vi "Event Handle Loop_Mouse Down.vi"(8 "error in (no error)":errorcluster, 10 "Coords":T1, 11 "QMenu Class in":refnum<class "QMenu Class.lvclass">) -> (0 "error out":errorcluster, 3 "QMenu Class out":refnum<class "QMenu Class.lvclass">)   [LabVIEW 2020, in "QTab.lvlib" / "QMenu Class.lvclass"]
uses:
  QMenu Class.lvclass
  <vilib>/Utility/miscctls.llb/LVPoint32TypeDef.ctl
  QMenu Class.lvclass/QMenu Class.ctl
  Read Total Button Count.vi
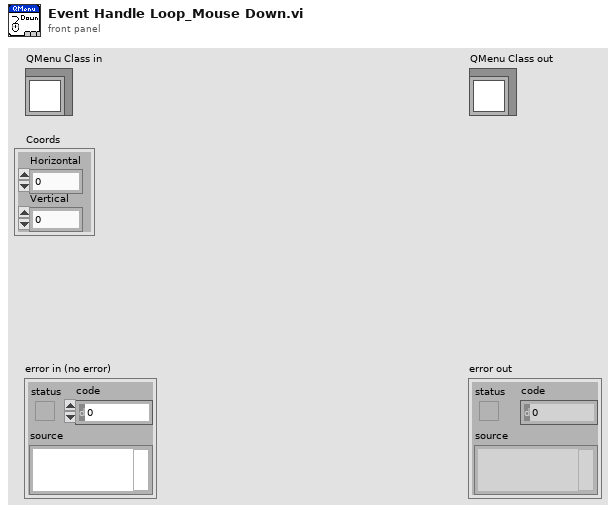
[diagram p1: front panel]
types:
  T1 = typedef "LVPoint32TypeDef.ctl" = cluster{"Horizontal":i32, "Vertical":i32}
  T2 = typedef "QTab.lvlib/QMenu Class.lvclass/Button Attribute.ctl" = cluster{"Label":string, "Button Text":string, "Closable":bool, "Draggable":bool}
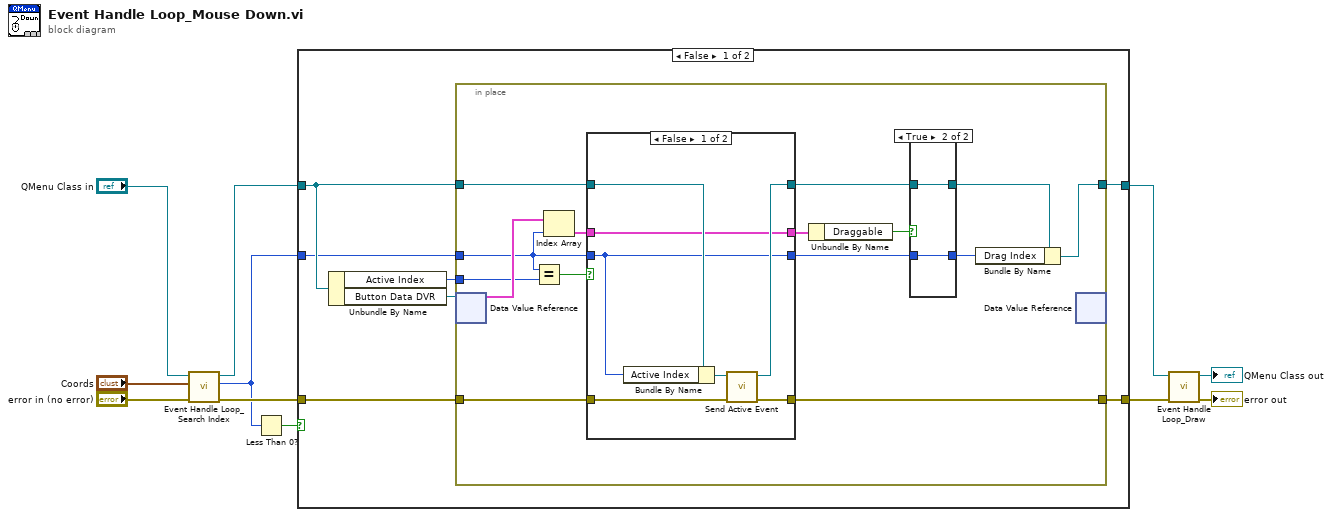
[diagram p0: block diagram]
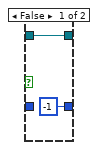
[diagram p2: hidden frame]
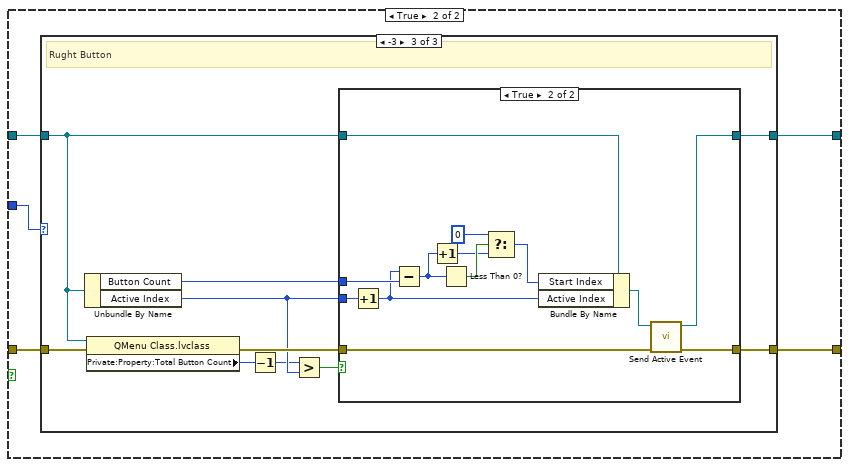
[diagram p4: hidden frame]
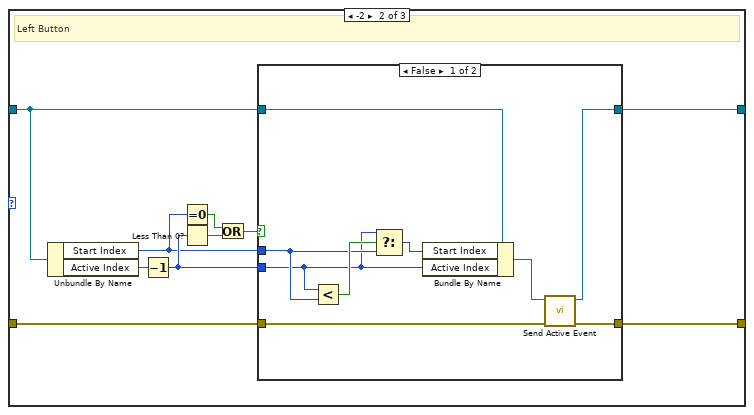
[diagram p6: hidden frame]
diagram:
  n1 = call "Event Handle Loop_Search Index.vi"("error in (no error)"="error in (no error)", "Coords"="Coords", "QMenu Class in"="QMenu Class in") -> ("error out"=w11:errorcluster, "Index"=w9:i32, "QMenu Class out"=w2:refnum<class "QMenu Class.lvclass">)  [unwired: 6 in]
  n2 = Less Than 0?(x=w9) -> (x < 0?=w3:bool)
  n3 = case shown="False" w3 {
    tunnel: w2 -> [w17 w51]
    tunnel: w9 -> [w13 w52]
    tunnel: [w14 w49] -> w1
    tunnel: w11 -> [w18 w53]
    tunnel: [w16 w50] -> w6
    frame False {
      n4 = Unbundle By Name(w17) -> ("Active Index"=w12:i32, "Button Data DVR"=w15:refnum<data-value>)
      n5 = in-place {
        in-place-border: w13 -> [w25]
        in-place-border: w18 -> [w33]
        in-place-border: w17 -> [w31]
        in-place-border: [w22] -> w16
        in-place-border: [w19] -> w14
        in-place-border: w12 -> [w24]
        n6 = in-place-dvr #1(w15) -> (w30:T2[])  [unwired: 1 out]
        n7 = Equal?(x=w25, y=w24) -> (x = y?=w32:bool)
        n8 = Index Array(array=w30, index=w25) -> (element=w29:T2)
        n9 = case shown="False" w32 {
          tunnel: w33 -> [w43 w48]
          tunnel: w31 -> [w44 w47]
          tunnel: [w40 w47] -> w26
          tunnel: [w41 w48] -> w22
          tunnel: w29 -> [w39 w46]
          tunnel: [w39 w46] -> w28
          tunnel: w25 -> [w38 w45]
          tunnel: [w38 w45] -> w23
          frame False {
            n10 = Bundle By Name(cluster=w44, "Active Index"=w38) -> (w42:refnum<class "QMenu Class.lvclass">)
            n11 = call "Send Active Event.vi"("error in (no error)"=w43, "QMenu Class in"=w42) -> ("error out"=w41:errorcluster, "QMenu Class out"=w40:refnum<class "QMenu Class.lvclass">)  [unwired: 8 in]
          }
          frame True {
          }
        }
        n12 = Unbundle By Name(w28) -> ("Draggable"=w27:bool)
        n13 = case shown="True" w27 {
          tunnel: w26 -> [w35 w36]
          tunnel: [w35 w36] -> w21
          tunnel: w23 -> [_ w37]
          tunnel: [-1 ("Index") w37] -> w20
          frame False {
          }
          frame True {
          }
        }
        n14 = Bundle By Name(cluster=w21, "Drag Index"=w20) -> (w19:refnum<class "QMenu Class.lvclass">)
        n15 = in-place-dvr #1() -> ()  [unwired: 1 in, 2 out]
      }
    }
    frame True {
      n16 = case shown="-3" w52 {
        tunnel: w53 -> [w54 w64 w86]
        tunnel: w51 -> [w55 w65 w83]
        tunnel: [w54 w63 w79] -> w50
        tunnel: [w55 w62 w82] -> w49
        frame Default {
        }
        frame -2 {
          # "Left Button"
          n17 = Unbundle By Name(w65) -> ("Start Index"=w59:i32, "Active Index"=w61:i32)
          n18 = Decrement(x=w61) -> (x-1=w60:i32)
          n19 = Equal To 0?(x=w59) -> (x = 0?=w57:bool)
          n20 = Less Than 0?(x=w60) -> (x < 0?=w58:bool)
          n21 = Or(x=w57, y=w58) -> (x .or. y?=w56:bool)
          n22 = case shown="False" w56 {
            tunnel: w65 -> [w74 w75]
            tunnel: w64 -> [w73 w76]
            tunnel: [w70 w76] -> w63
            tunnel: [w71 w75] -> w62
            tunnel: w60 -> [w66 _]
            tunnel: w59 -> [w68 _]
            frame False {
              n23 = Less?(x=w66, y=w68) -> (x < y?=w69:bool)
              n24 = Select(t=w66, s=w69, f=w68) -> (s? t:f=w67:i32)
              n25 = Bundle By Name(cluster=w74, "Start Index"=w67, "Active Index"=w66) -> (w72:refnum<class "QMenu Class.lvclass">)
              n26 = call "Send Active Event.vi"("error in (no error)"=w73, "QMenu Class in"=w72) -> ("error out"=w70:errorcluster, "QMenu Class out"=w71:refnum<class "QMenu Class.lvclass">)  [unwired: 8 in]
            }
            frame True {
            }
          }
        }
        frame -3 {
          # "Rught Button"
          n27 = Unbundle By Name(w83) -> ("Button Count"=w80:i32, "Active Index"=w81:i32)
          n28 = property class="QMenu Class.lvclass"(reference=w83, error in=w86) -> (error out=w84:errorcluster, "Private:Property:Total Button Count"=w78:i32)  [unwired: 1 out]
          n29 = Decrement(x=w78) -> (x-1=w77:i32)
          n30 = Greater?(x=w77, y=w81) -> (0:w85:bool)
          n31 = case shown="True" w85 {
            tunnel: w84 -> [w87 w92]
            tunnel: w83 -> [w88 w100]
            tunnel: [w88 w90] -> w82
            tunnel: w81 -> [_ w101]
            tunnel: w80 -> [_ w99]
            tunnel: [w87 w89] -> w79
            frame False {
            }
            frame True {
              n32 = Increment(x=w101) -> (x+1=w96:i32)
              n33 = Subtract(x=w96, y=w99) -> (x-y=w93:i32)
              n34 = Increment(x=w93) -> (x+1=w95:i32)
              n35 = Less Than 0?(x=w93) -> (x < 0?=w98:bool)
              n36 = Select(t=0, s=w98, f=w95) -> (s? t:f=w94:i32)
              n37 = Bundle By Name(cluster=w100, "Start Index"=w94, "Active Index"=w96) -> (w91:refnum<class "QMenu Class.lvclass">)
              n38 = call "Send Active Event.vi"("error in (no error)"=w92, "QMenu Class in"=w91) -> ("error out"=w89:errorcluster, "QMenu Class out"=w90:refnum<class "QMenu Class.lvclass">)  [unwired: 8 in]
            }
          }
        }
      }
    }
  }
  n39 = call "Event Handle Loop_Draw.vi"("error in (no error)"=w6, "QMenu Class in"=w1) -> ("error out"=→"error out":errorcluster, "QMenu Class out"=→"QMenu Class out":refnum<class "QMenu Class.lvclass">)  [unwired: 8 in]
